vi "Intan_VerifySerialLink.vi"(8 "error in":errorcluster, 11 "VISA resource name":refnum<visa-resource-name>="COM1") -> (0 "error out":errorcluster, 2 "verifySpiResponse":string, 3 "VISA resource name out":refnum<visa-resource-name>)   [LabVIEW 2020]
panel:
  out "return count spi1":u32
  out "verify Spi1":string
  in  "bytes to read":u32=1000
  out "return count":u32
  out "verifySpi0":string
  in  "Teensy event char":string="v"
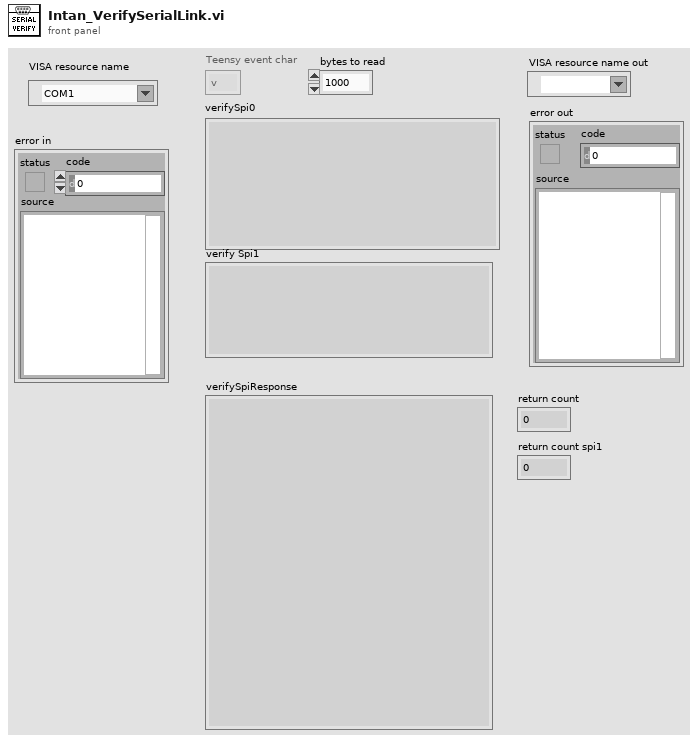
[diagram p1: front panel]
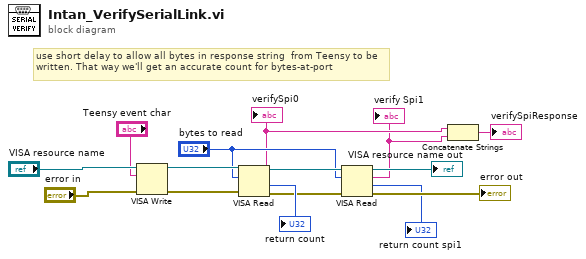
[diagram p0: block diagram]
diagram:
  # "use short delay to allow all bytes in response string  from Teensy to be written. That way we'll get an accurate count for bytes-at-port"
  n1 = VISA Write(VISA resource name="VISA resource name", write buffer="Teensy event char", error in (no error)="error in") -> (VISA resource name out=w12:refnum<visa-resource-name>, error out=w11:errorcluster)  [unwired: 1 out]
  n2 = VISA Read(VISA resource name=w12, byte count="bytes to read", error in (no error)=w11) -> (VISA resource name out=w9:refnum<visa-resource-name>, read buffer=w3:string, return count=→"return count":u32, error out=w8:errorcluster)
  "verifySpi0" <- w3
  n3 = VISA Read(VISA resource name=w9, byte count="bytes to read", error in (no error)=w8) -> (VISA resource name out=→"VISA resource name out":refnum<visa-resource-name>, read buffer=w2:string, return count=→"return count spi1":u32, error out=→"error out":errorcluster)
  "verify Spi1" <- w2
  n4 = Concatenate Strings(w3, w2) -> (→"verifySpiResponse":string)
